vi "JL_LED Translation.vi"(7 "Model Select":T8, 8 "error in (no error)":errorcluster, 10 "Option":T9, 11 "JL Display":T1={"SSD"="", "Cycle Selection"=enum."Cycle 0", "Bar Selection"=enum."Bar 1", "Temp Setting"=enum."High", "Dryness Level"=enum."Extra Dry", "Time Setting"=enum."Default Time 5", "Dryer Status"=enum."Status 6", "Start/Pause"=FALSE, "Pause"=FALSE, "Control Lock"=FALSE, "Sensing"=FALSE, "Clean Filter"=FALSE, "My Cycle"=FALSE, "Delay Dry"=FALSE, "Volume"=FALSE, "Damp Alert"=FALSE, "Ext Tumble"=FALSE, "Decrement"=FALSE, "Increment"=FALSE, "eDry"=FALSE, "Extra Status"=FALSE}) -> (0 "error out":errorcluster, 3 "JL Display 2":T1={"SSD"="", "Cycle Selection"=enum."Cycle 0", "Bar Selection"=enum."Bar 1", "Temp Setting"=enum."High", "Dryness Level"=enum."Extra Dry", "Time Setting"=enum."Default Time 5", "Dryer Status"=enum."Status 6", "Start/Pause"=FALSE, "Pause"=FALSE, "Control Lock"=FALSE, "Sensing"=FALSE, "Clean Filter"=FALSE, "My Cycle"=FALSE, "Delay Dry"=FALSE, "Volume"=FALSE, "Damp Alert"=FALSE, "Ext Tumble"=FALSE, "Decrement"=FALSE, "Increment"=FALSE, "eDry"=FALSE, "Extra Status"=FALSE})   [LabVIEW 2016]
uses:
  type defs/JL Display.ctl
  type defs/Cycle Selection Enum.ctl
  type defs/Bar Enum.ctl
  type defs/Temp Setting Enum.ctl
  type defs/Dryness Enum.ctl
  type defs/Time Enum.ctl
  type defs/Status Enum.ctl
  type defs/JL_Trans-state.ctl
  type defs/JL_Trans-Model.ctl
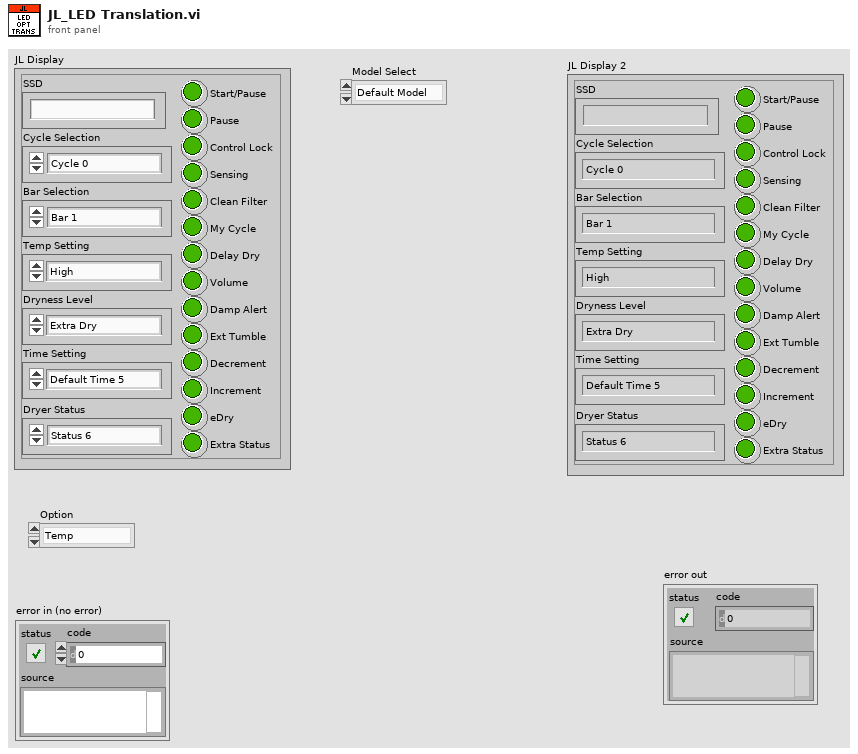
[diagram p1: front panel]
types:
  T1 = typedef "JL Display.ctl" = cluster{"SSD":string, "Cycle Selection":T2, "Bar Selection":T3, "Temp Setting":T4, "Dryness Level":T5, "Time Setting":T6, "Dryer Status":T7, "Start/Pause":bool, "Pause":bool, "Control Lock":bool, "Sensing":bool, "Clean Filter":bool, "My Cycle":bool, "Delay Dry":bool, "Volume":bool, "Damp Alert":bool, "Ext Tumble":bool, "Decrement":bool, "Increment":bool, "eDry":bool, "Extra Status":bool}
  T2 = typedef "Cycle Selection Enum.ctl" = enum16{"Cycle 0", "Cycle 1", "Cycle 2", "Cycle 3", "Cycle 4", "Cycle 5", "Cycle 6", "Cycle 7", "Cycle 8", "Cycle 9", "Cycle 10", "Cycle 11", "Cycle 12", "Cycle 13", "Off", "*Invalid"}
  T3 = typedef "Bar Enum.ctl" = enum16{"Bar 1", "Bar 2", "Bar 3", "Bar 4", "Bar 5", "Off", "*Incorrect*"}
  T4 = typedef "Temp Setting Enum.ctl" = enum16{"Off", "No Heat", "Extra Low", "Low", "Medium", "High", "*Incorrect*"}
  T5 = typedef "Dryness Enum.ctl" = enum16{"Off", "Damp", "Less Dry", "Dry", "More Dry", "Extra Dry", "*Incorrect*"}
  T6 = typedef "Time Enum.ctl" = enum16{"Off", "Default Time 1", "Default Time 2", "Default Time 3", "Default Time 4", "Default Time 5", "*Incorrect*"}
  T7 = typedef "Status Enum.ctl" = enum16{"Status 1", "Status 2", "Status 3", "Status 4", "Status 5", "Status 6", "Off", "*Incorrect*"}
  T8 = typedef "JL_Trans-Model.ctl" = enum16{"Default Model"}
  T9 = typedef "JL_Trans-state.ctl" = enum16{"Temp ", "Time", "Level", "stop"}
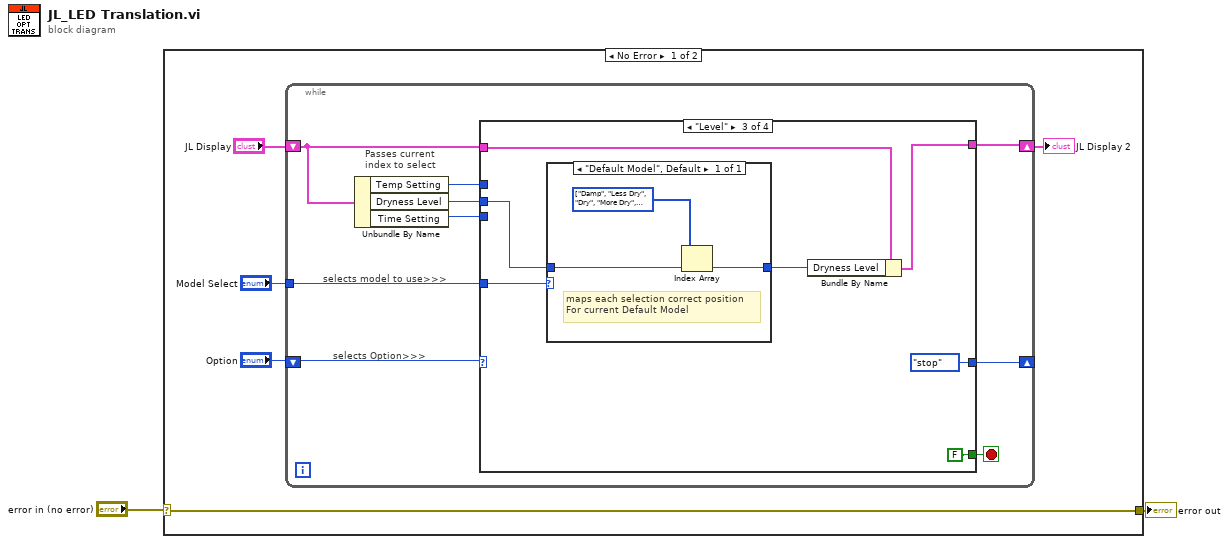
[diagram p0: block diagram]
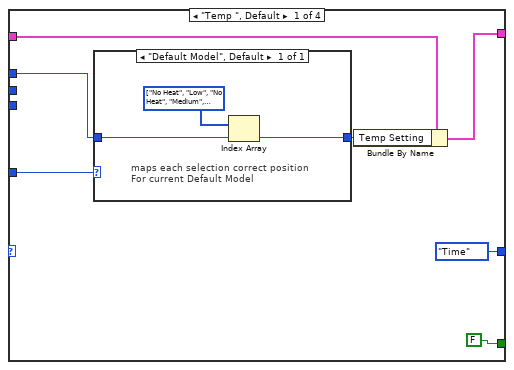
[diagram p2: hidden frame]
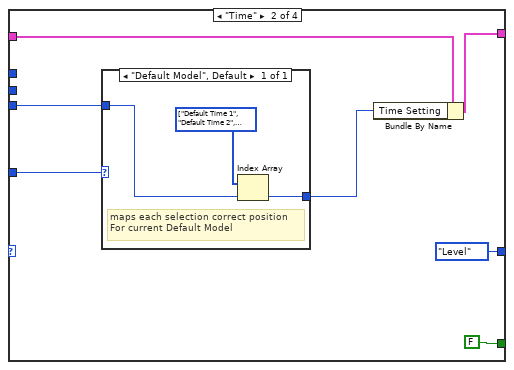
[diagram p3: hidden frame]
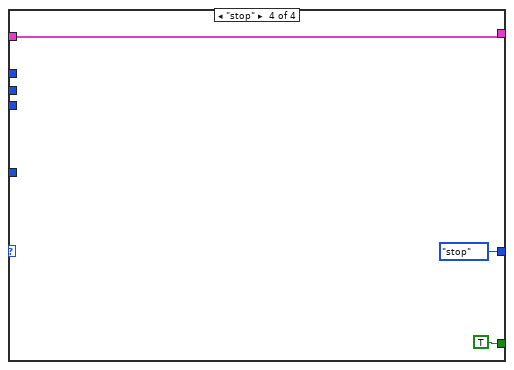
[diagram p4: hidden frame]
diagram:
  n1 = case shown="No Error" "error in (no error)" {
    selector: "error in (no error)" -> [w4 w50]
    tunnel: [w4 w50] -> w1
    frame No Error {
      n2 = while {
        shift-right: [w14] -> w3
        shift-left: "JL Display" -> [w13]
        tunnel: "Model Select" -> [w9]
        shift-right: [w8] -> _
        shift-left: "Option" -> [w16]
        stop <- w15 stop-if-true
        # "Passes current \nindex to select"
        # "selects Option>>>"
        # "selects model to use>>>"
        n3 = Unbundle By Name(w13) -> ("Temp Setting"=w12:T4, "Dryness Level"=w10:T5, "Time Setting"=w11:T6)
        n4 = case shown="\"Level\"" w16 {
          tunnel: [FALSE FALSE FALSE TRUE] -> w15
          tunnel: w13 -> [w22 w32 w42 w48]
          tunnel: [w21 w31 w41 w48] -> w14
          tunnel: w12 -> [w20 _ _ _]
          tunnel: w11 -> [_ w29 _ _]
          tunnel: w10 -> [_ _ w38 _]
          tunnel: w9 -> [w18 w30 w39 _]
          tunnel: [JL_Trans-state."Time" ("Enum") JL_Trans-state."Level" ("Enum") JL_Trans-state."stop" ("Enum") JL_Trans-state."stop" ("Enum")] -> w8
          frame "Temp ", Default {
            n5 = case shown="\"Default Model\", Default" w18 {
              tunnel: [w26] -> w19
              tunnel: w20 -> [w25]
              frame "Default Model", Default {
                w24 = T4[] [enum."No Heat", enum."Low", enum."No Heat", enum."Medium", enum."High"] items=["Off", "No Heat", "Extra Low", "Low", "Medium", "High", "*Incorrect*"]
                # "maps each selection correct position\nFor current Default Model"
                n6 = Index Array(array=w24, index=w25) -> (element=w26:T4)
              }
            }
            n7 = Bundle By Name(cluster=w22, "Temp Setting"=w19) -> (w21:T1)
          }
          frame "Time" {
            n8 = case shown="\"Default Model\", Default" w30 {
              tunnel: w29 -> [w35]
              tunnel: [w34] -> w28
              frame "Default Model", Default {
                w36 = T6[] [enum."Default Time 1", enum."Default Time 2", enum."Default Time 3", enum."Default Time 4", enum."*Incorrect*", enum."Default Time 5", enum."Off"] items=["Off", "Default Time 1", "Default Time 2", "Default Time 3", "Default Time 4", "Default Time 5", "*Incorrect*"]
                # "maps each selection correct position\nFor current Default Model"
                n9 = Index Array(array=w36, index=w35) -> (element=w34:T6)
              }
            }
            n10 = Bundle By Name(cluster=w32, "Time Setting"=w28) -> (w31:T1)
          }
          frame "Level" {
            n11 = case shown="\"Default Model\", Default" w39 {
              tunnel: [w46] -> w40
              tunnel: w38 -> [w44]
              frame "Default Model", Default {
                w45 = T5[] [enum."Damp", enum."Less Dry", enum."Dry", enum."More Dry", enum."Off"] items=["Off", "Damp", "Less Dry", "Dry", "More Dry", "Extra Dry", "*Incorrect*"]
                # "maps each selection correct position\nFor current Default Model"
                n12 = Index Array(array=w45, index=w44) -> (element=w46:T5)
              }
            }
            n13 = Bundle By Name(cluster=w42, "Dryness Level"=w40) -> (w41:T1)
          }
          frame "stop" {
          }
        }
      }
      "JL Display 2" <- w3
    }
    frame Error {
    }
  }
  "error out" <- w1
